vi "Configure Gate View (Bandwidth).vi"(0 "VISA resource name":refnum<visa-resource-name>, 5 "Auto Resolution Gate View BW(T:Enable)":bool=TRUE, 7 "Resolution Gate View BW (6:30kHz)":i32(ring)=6 items=["30 Hz", "100 Hz", "300 Hz", "1 kHz", "3 kHz", "10 kHz", "30 kHz", "50 kHz", "100 kHz", "300 kHz", "1 MHz", "3 MHz", "5 MHz", "10 MHz", "20 MHz", "31.25 MHz"], 9 "Auto Video Gate View BW (T:Enable)":bool=TRUE, 11 "error in (no error)":errorcluster, 12 "Video Gate View BW (0:Off)":i32(ring) items=["Off", "1 Hz", "3 Hz", "10 Hz", "30 Hz", "100 Hz", "300 Hz", "1 kHz", "3 kHz", "5 kHz", "10 kHz", "30 kHz", "100 kHz", "300 kHz", "1 MHz", "3 MHz", "10 MHz"]) -> (4 "VISA resource name out":refnum<visa-resource-name>, 15 "error out":errorcluster)   [LabVIEW 2020, in "Anritsu Signal Analyzer Series.lvlib"]
doc: "Configures the gate view (Bandwidth) settings of the spectrum analyzer."
uses:
  Anritsu Signal Analyzer Series.lvlib
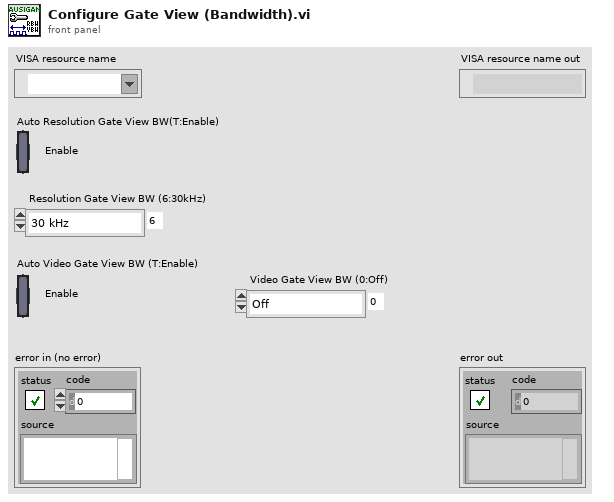
[diagram p1: front panel]
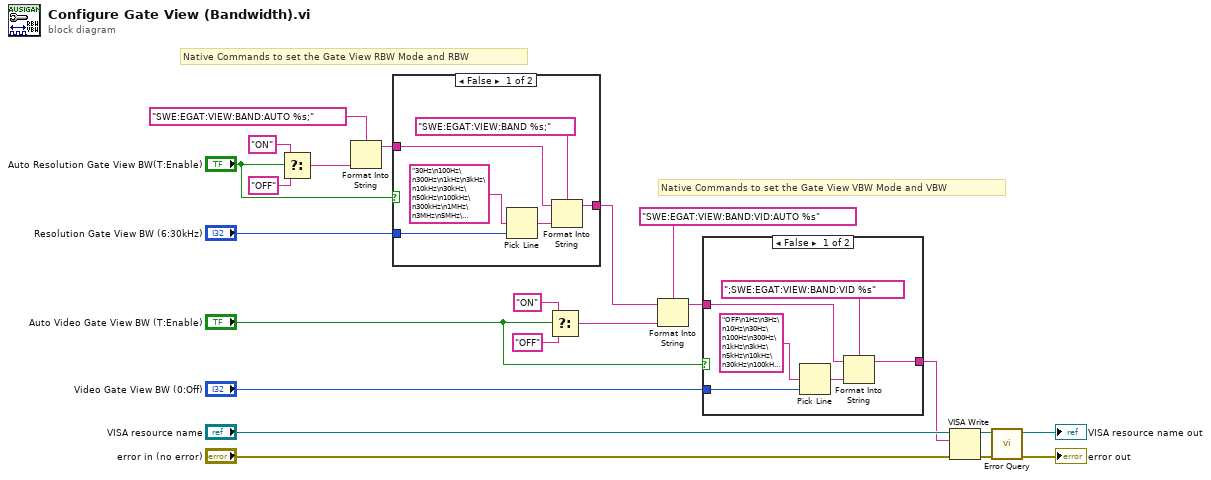
[diagram p0: block diagram]
diagram:
  # "Native Commands to set the Gate View VBW Mode and VBW"
  # "Native Commands to set the Gate View RBW Mode and RBW"
  n1 = Select(t="ON" ("string"), s="Auto Resolution Gate View BW(T:Enable)", f="OFF" ("string")) -> (s? t:f=w6:string)
  n2 = Format Into String(format string="SWE:EGAT:VIEW:BAND:AUTO %s;" ("_CommandSet"), w6) -> (resulting string=w15:string)  [unwired: 2 in, 1 out]
  n3 = case shown="False" "Auto Resolution Gate View BW(T:Enable)" {
    tunnel: "Resolution Gate View BW (6:30kHz)" -> [w23 _]
    tunnel: w15 -> [w27 w29]
    tunnel: [w26 w29] -> w13
    frame False {
      n4 = Pick Line(multi-line string="30Hz\n100Hz\n300Hz\n1kHz\n3kHz\n10kHz\n30kHz\n50kHz\n100kHz\n300kHz\n1MHz\n3MHz\n5MHz\n10MHz\n20MHz\n31.25MHz" ("文字列"), line index=w23) -> (output string=w24:string)  [unwired: 1 in]
      n5 = Format Into String(format string="SWE:EGAT:VIEW:BAND %s;" ("_CommandSet"), initial string=w27, w24) -> (resulting string=w26:string)  [unwired: 1 in, 1 out]
    }
    frame True {
    }
  }
  n6 = Select(t="ON" ("string"), s="Auto Video Gate View BW (T:Enable)", f="OFF" ("string")) -> (s? t:f=w3:string)
  n7 = Format Into String(format string="SWE:EGAT:VIEW:BAND:VID:AUTO %s" ("_CommandSet"), initial string=w13, w3) -> (resulting string=w12:string)  [unwired: 1 in, 1 out]
  n8 = case shown="False" "Auto Video Gate View BW (T:Enable)" {
    tunnel: "Video Gate View BW (0:Off)" -> [w31 _]
    tunnel: w12 -> [w34 w36]
    tunnel: [w33 w36] -> w9
    frame False {
      n9 = Pick Line(multi-line string="OFF\n1Hz\n3Hz\n10Hz\n30Hz\n100Hz\n300Hz\n1kHz\n3kHz\n5kHz\n10kHz\n30kHz\n100kHz\n300kHz\n1MHz\n3MHz\n10MHz" ("文字列"), line index=w31) -> (output string=w32:string)  [unwired: 1 in]
      n10 = Format Into String(format string=";SWE:EGAT:VIEW:BAND:VID %s" ("_CommandSet"), initial string=w34, w32) -> (resulting string=w33:string)  [unwired: 1 in, 1 out]
    }
    frame True {
    }
  }
  n11 = VISA Write(VISA resource name="VISA resource name", write buffer=w9, error in (no error)="error in (no error)") -> (VISA resource name out=w11:refnum<visa-resource-name>, error out=w10:errorcluster)  [unwired: 1 out]
  n12 = call "Error Query.vi"("error in (no error)"=w10, "VISA resource name"=w11) -> ("error out"=→"error out":errorcluster, "VISA resource name out"=→"VISA resource name out":refnum<visa-resource-name>)  [unwired: 6 in, 2 out]
